vi "Write Command Name.vi"(8 "error in (no error)":errorcluster, 10 "Command Name":string, 11 "Command in":refnum<class "Command Actor.lvclass">) -> (0 "error out":errorcluster, 3 "Command out":refnum<class "Command Actor.lvclass">)   [LabVIEW 2014, in "Robot Actor Framework.lvlib" / "Command Actor.lvlib" / "Command Actor.lvclass"]
uses:
  Command Actor.lvclass
  Command Actor.lvclass/Command Actor.ctl
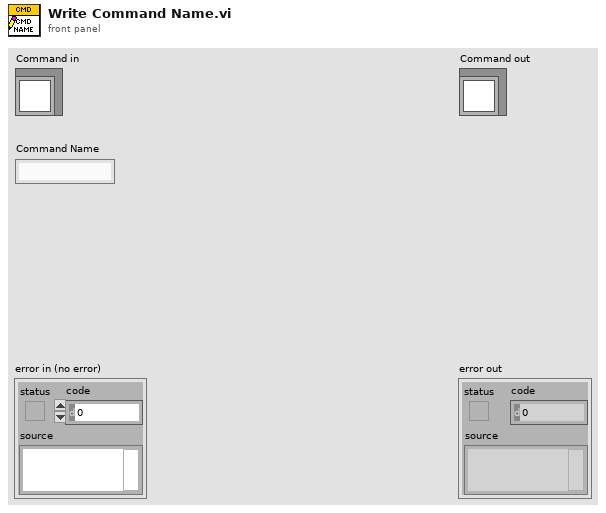
[diagram p1: front panel]
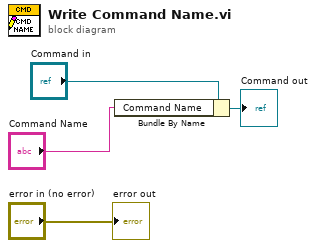
[diagram p0: block diagram]
diagram:
  n1 = Bundle By Name(cluster="Command in", "Command Name"="Command Name") -> (→"Command out":refnum<class "Command Actor.lvclass">)
  "error out" <- "error in (no error)"
